vi "Create NetworkHandler.vi"(7 "Formatter.lvclass":refnum<class "Formatter.lvclass">, 8 "error in":errorcluster, 9 "Level":T1, 10 "Name":string, 11 "NetworkHandler in":refnum<class "INetworkWriter.lvclass">) -> (0 "error out":errorcluster, 3 "NetworkHandler out":refnum<class "StreamLogHandle.lvclass">)   [LabVIEW 2024, in "StreamLogHandle.lvclass"]
doc: "Creates and initializes a new FileHandler object.\n\n____\nHAMPEL SOFTWARE ENGINEERING v2.2.2 (2025-01-16 15:41)"
uses:
  StreamLogHandle.lvclass
  StreamLogHandle.lvclass/StreamLogHandle.ctl
  <vilib>/Hampel Software Engineering/HSE Logger/LogLevel.ctl
  <vilib>/Hampel Software Engineering/HSE Logger/hse-logger.lvlib
  <vilib>/Hampel Software Engineering/HSE Logger/Formatter/Formatter.lvclass
  Stream/INetworkWriter/INetworkWriter.lvclass
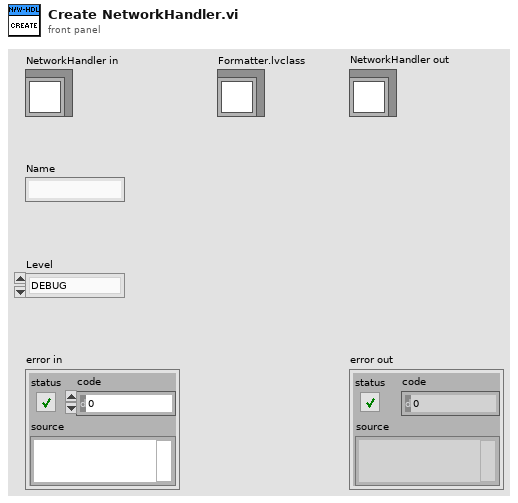
[diagram p1: front panel]
types:
  T1 = typedef "hse-logger.lvlib/LogLevel.ctl" = enum16{"DEBUG", "INFO", "WARNING", "ERROR", "CRITICAL"}
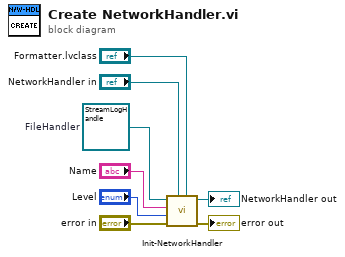
[diagram p0: block diagram]
diagram:
  w8 = refnum<class "StreamLogHandle.lvclass"> refnum  # FileHandler
  n1 = call-dynamic "Init-NetworkHandler.vi"("Formatter.lvclass"="Formatter.lvclass", "INetworkWriter"="NetworkHandler in", "error in"="error in", "Level"="Level", "Name"="Name", "NetworkHandler in"=w8) -> ("error out"=→"error out":errorcluster, "NetworkHandler out"=→"NetworkHandler out":refnum<class "StreamLogHandle.lvclass">)  [unwired: 4 in]
